vi "Butterfly_PullUp Capacitance AWG.vi"(0 "Semiconductor Module Context":T2, 2 "script name":string, 3 "C_TH_Delta":dbl=0.03 format="%#_13g", 4 "VNAs Measurement Parameters":T1, 5 "error in (no error)":errorcluster, 9 "Start_v":dbl=10.0 format="%#_13g", 11 "Stop_v":dbl=41.0 format="%#_13g") -> (14 "Semiconductor Module Context Out":T2, 19 "error out":errorcluster)   [LabVIEW 2013]
uses:
  <vilib>/NI_TestStand_SemiconductorModule/NI_TestStand_Semiconductor_Module.lvlibp/PinMap/General/SemiconductorModuleContext.ctl
  VNA/VNAs Measurement Parameters.ctl
  <instrlib>/niDCPower/nidcpower.llb/niDCPower Wait For Event - Event.ctl
  <instrlib>/niHSDIO/niHSDIO.llb/niHSDIO_ctl Trigger Script - trigID Values (Ring).ctl
  <vilib>/NI_TestStand_SemiconductorModule/NI_TestStand_Semiconductor_Module.lvlibp/PinMap/General/Publish/PublishDataDouble2D.vi
  <vilib>/NI_TestStand_SemiconductorModule/NI_TestStand_Semiconductor_Module.lvlibp
  VNA/Pin Map API/VNA Custom Instrument.lvlib
panel:
  out "Site":i32
  out "RL Step":i32
  out "PI Step":i32
  out "C_TH_PU":dbl format="%#_3g"
  out "C_Free":dbl[](array[numeric]) format="%#_3g"
  out "max index":i32
  out "BF C PI":dbl format="%#_3g"
  out "C_VPI":dbl
  out "BF C RL":dbl format="%#_3g"
  out "C_VRL":dbl
  out "appended array":dbl[][](array[numeric]) format="%#_3g"
  out "S3 steps":dbl[](array[numeric]) format="%#_3g"
  out "S2 steps":dbl[](array[numeric]) format="%#_3g"
  out "S1 steps":dbl[](array[numeric]) format="%#_3g"
  out "S0 steps":dbl[](array[numeric]) format="%#_3g"
  out "BF values":dbl[](array[numeric])
  out "VRLs":dbl[](array[numeric])
  out "VPIs":dbl[](array[numeric])
  out "Multisite Cap Data":dbl[][][](array[numeric])
  out "BF Names":string[](array[string])
  out "BFSamples":i32
  in  "Step_v":dbl=1.0
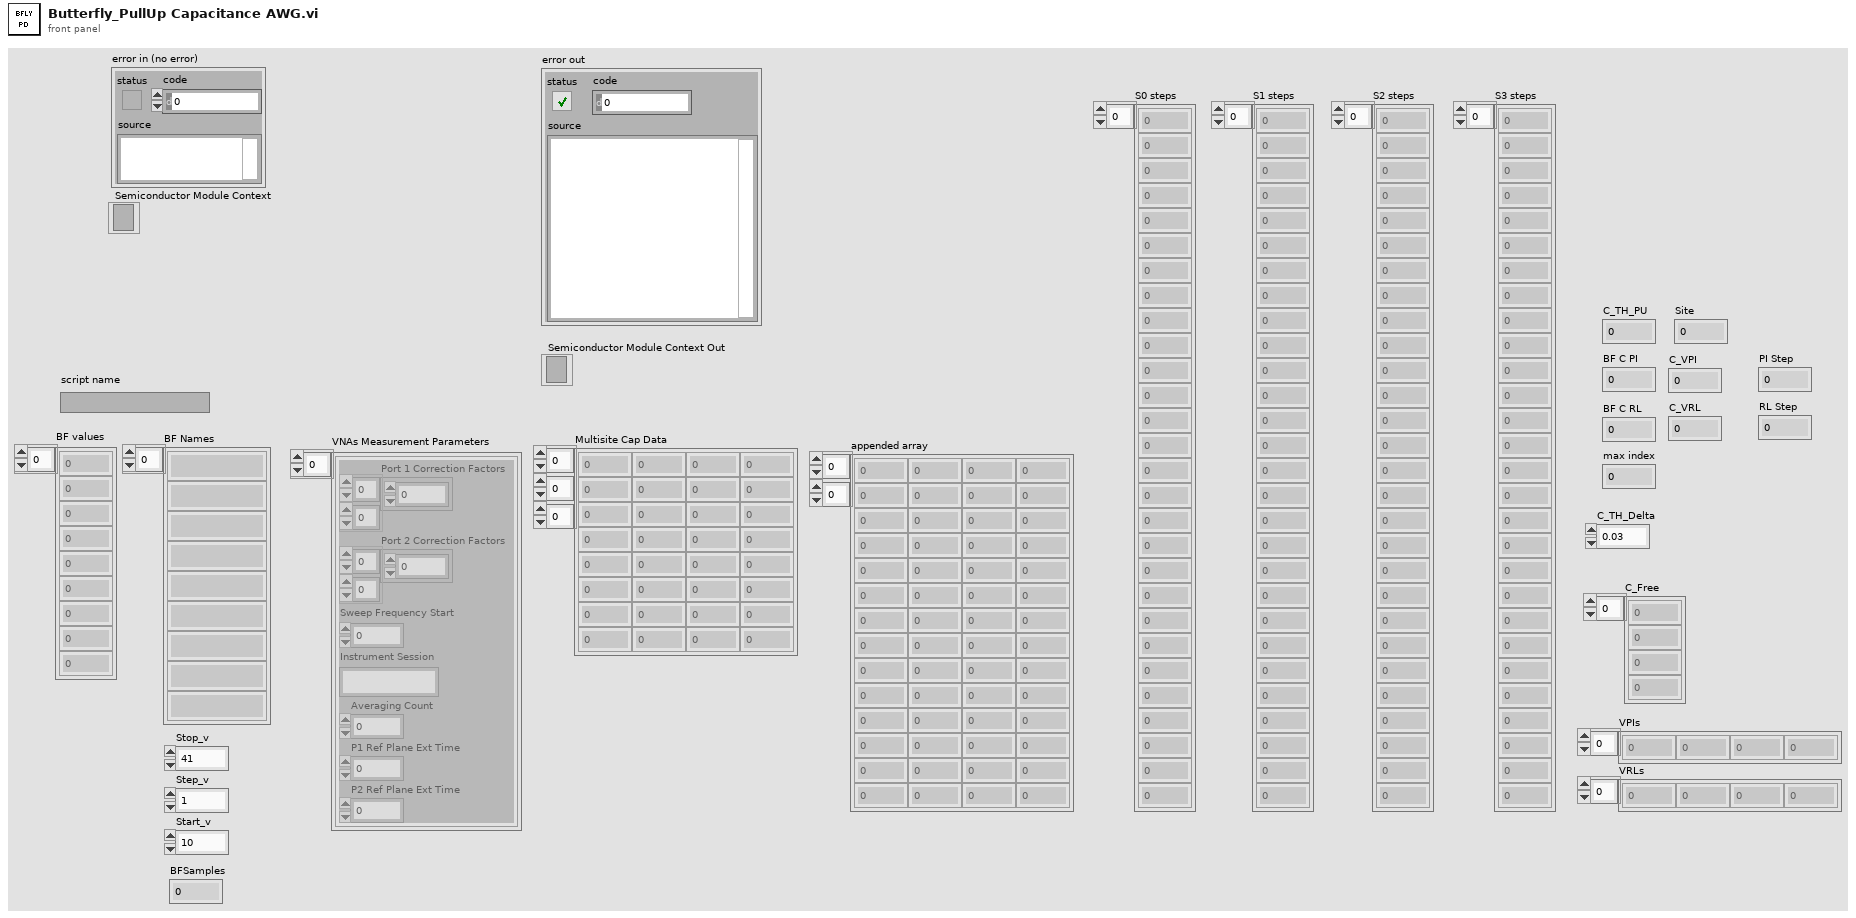
[diagram p1: front panel]
types:
  T1 = typedef "VNAs Measurement Parameters.ctl" = cluster{"Port 1 Correction Factors":cdb[][], "Port 2 Correction Factors":cdb[][], "Sweep Frequency Start":dbl, "Instrument Session":string, "Averaging Count":i32, "P1 Ref Plane Ext Time":dbl, "P2 Ref Plane Ext Time":dbl}[]
  T2 = typedef "NI_TestStand_Semiconductor_Module.lvlibp/SemiconductorModuleContext.ctl" = refnum<k7>
  T3 = typedef "niHSDIO_ctl Trigger Script - trigID Values (Ring).ctl" = string
  T4 = typedef "niDCPower Wait For Event - Event.ctl" = i32
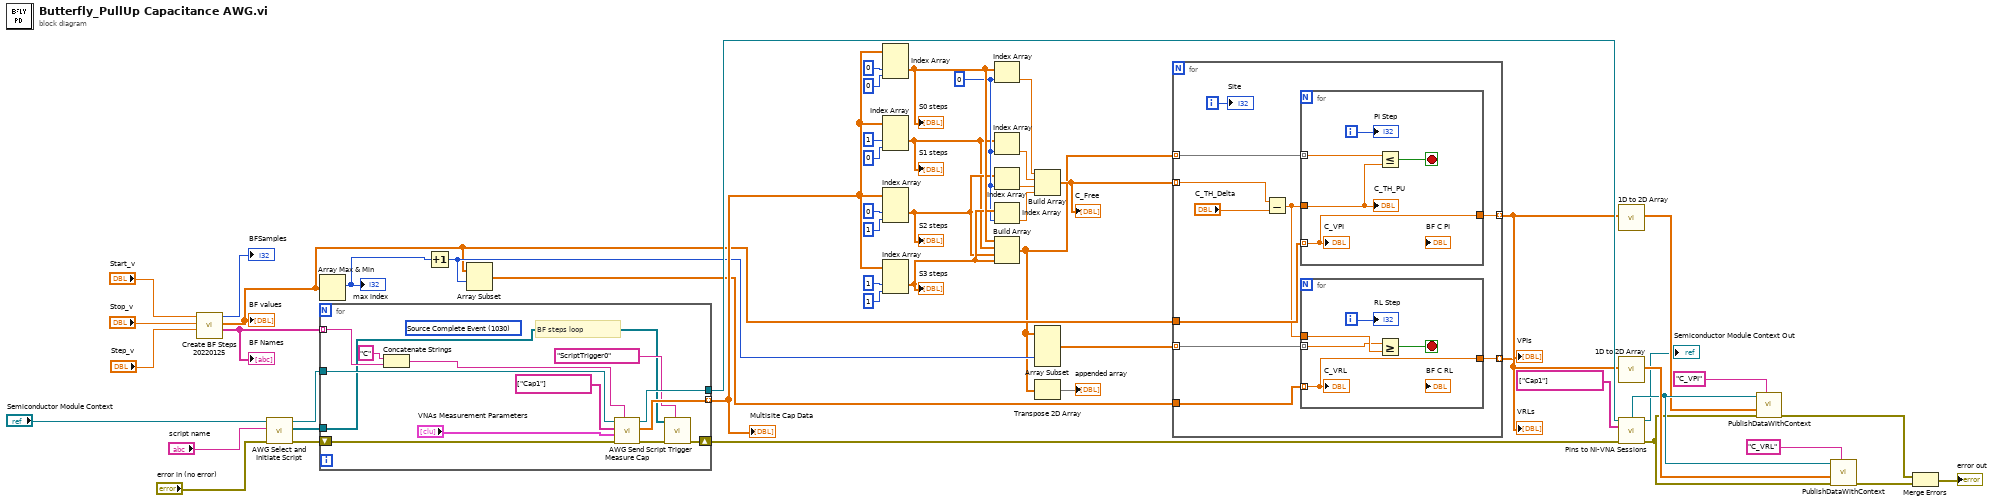
[diagram p0: block diagram]
diagram:
  w16 = 0 ("index")
  n1 = call "Create BF Steps 20220125.vi"("Step_v"="Step_v", "Stop_v"="Stop_v", "Start_v"="Start_v") -> ("BF Names"=w47:string[], "BF values"=w23:dbl[], "BFSamples"=→"BFSamples":i32)  [unwired: 6 in]
  "BF Names" <- w47
  "BF values" <- w23
  n2 = call "AWG Select and Initiate Script.vi"("error in (no error)"="error in (no error)", "script name"="script name", "Semiconductor Module Context"="Semiconductor Module Context") -> ("error out"=w2:errorcluster, "Sessions Out"=w6:refnum<k15>[], "Semiconductor Module Context Out"=w1:T2)  [unwired: 6 in]
  n3 = Array Max & Min(array=w23) -> (max index (indices)=w25:i32)  [unwired: 3 out]
  "max index" <- w25
  n4 = for {
    shift-right: [w55] -> w45
    shift-left: w2 -> [w57]
    tunnel: w1 -> [w62]
    tunnel: [w61] -> w52
    tunnel: [w60] -> w46 mode=indexing
    tunnel: w47 -> [w64] mode=indexing
    tunnel: w6 -> [w53]
    (unwired) T4 1030 items=["Source Complete Event"=1030, "Measure Complete Event"=1031, "Sequence Iteration Complete Event"=1032, "Sequence Engine Done Event"=1033, "Pulse Complete Event"=1051, "Ready For Pulse Trigger Event"=1052] ("event")
    # "BF steps loop"
    n5 = Concatenate Strings("C" ("string"), w64) -> (w63:string)
    n6 = call "Measure Cap.vi"("Measurement Id"=w63, "error in (no error)"=w57, "VNAs Measurement Parameters"="VNAs Measurement Parameters", "Pins"=string[] ["Cap1"] ("Capacitance Pins"), "Semiconductor Module Context"=w62) -> ("error out"=w56:errorcluster, "Multisite Cap Data"=w60:dbl[][], "Semiconductor Module Context Out"=w61:T2)  [unwired: 4 in]
    n7 = call "AWG Send Script Trigger.vi"("trigger id (script trigger 0)"=T3 "ScriptTrigger0", "error in (no error)"=w56, "AWG Sessions In"=w53) -> ("error out"=w55:errorcluster)  [unwired: 7 in, 1 out]
  }
  "Multisite Cap Data" <- w46
  n8 = Increment(x=w25) -> (x+1=w24:i32)
  n9 = Array Subset(array=w23, index=w24) -> (w22:dbl[])  [unwired: 1 in]
  n10 = Index Array(array=w46, index (dim 1)=0 ("disabled index (row)"), index (dim 2)=0 ("disabled index (col)")) -> (element=w19:dbl[])  [unwired: 1 in]
  "S0 steps" <- w19
  n11 = Index Array(array=w46, index (dim 1)=1 ("index (row)"), index (dim 2)=0 ("index (col)")) -> (element=w10:dbl[])  [unwired: 1 in]
  "S1 steps" <- w10
  n12 = Index Array(array=w46, index (dim 1)=0 ("index (row)"), index (dim 2)=1 ("index (col)")) -> (element=w11:dbl[])  [unwired: 1 in]
  "S2 steps" <- w11
  n13 = Index Array(array=w46, index (dim 1)=1 ("index (row)"), index (dim 2)=1 ("index (col)")) -> (element=w17:dbl[])  [unwired: 1 in]
  "S3 steps" <- w17
  n14 = Index Array(array=w19, index=w16) -> (element=w18:dbl)
  n15 = Index Array(array=w10, index=w16) -> (element=w15:dbl)
  n16 = Index Array(array=w11, index=w16) -> (element=w13:dbl)
  n17 = Index Array(array=w17, index=w16) -> (element=w14:dbl)
  n18 = Build Array(w19, w10, w11, w17) -> (w9:dbl[][])
  n19 = Build Array(w18, w15, w13, w14) -> (w12:dbl[])
  "C_Free" <- w12
  n20 = Array Subset(array=w9, index (col)=w24) -> (w26:dbl[][])  [unwired: 3 in]
  n21 = Transpose 2D Array(2D array=w9) -> (transposed array=→"appended array":dbl[][])
  n22 = for {
    tunnel: w23 -> [w75]
    tunnel: [w74] -> w21 mode=indexing
    tunnel: w22 -> [w73]
    tunnel: w26 -> [w72] mode=indexing
    tunnel: [w71] -> w20 mode=indexing
    tunnel: w12 -> [w68] mode=indexing
    tunnel: w9 -> [w69] mode=indexing
    i -> [w70]
    n23 = Subtract(x=w68, y="C_TH_Delta") -> (x-y=w66:dbl)
    n24 = for {
      tunnel: w75 -> [w84] mode=indexing
      tunnel: [w84] -> w74
      tunnel: w66 -> [w83]
      tunnel: w69 -> [w81] mode=indexing
      i -> [w82]
      stop <- w85 stop-if-true
      n25 = Less Or Equal?(x=w81, y=w83) -> (x <= y?=w85:bool)
      "C_VPI" <- w84
      "C_TH_PU" <- w83
      "PI Step" <- w82
    }
    n26 = for {
      tunnel: w73 -> [w79] mode=indexing
      tunnel: w72 -> [w76] mode=indexing
      tunnel: [w79] -> w71
      tunnel: w66 -> [w78]
      i -> [w77]
      stop <- w80 stop-if-true
      n27 = Greater Or Equal?(x=w76, y=w78) -> (x >= y?=w80:bool)
      "C_VRL" <- w79
      "RL Step" <- w77
    }
    "Site" <- w70
  }
  "VPIs" <- w21
  "VRLs" <- w20
  n28 = call "1D to 2D Array.vi"("1D Array"=w21) -> ("2D Array"=w30:dbl[][])  [unwired: 10 in]
  n29 = call "1D to 2D Array.vi"("1D Array"=w20) -> ("2D Array"=w43:dbl[][])  [unwired: 10 in]
  n30 = call "Pins to NI-VNA Sessions.vi"("Semiconductor Module Context"=w52, "Pins"=string[] ["Cap1"] ("Capacitance Pins"), "error in (no error)"=w45) -> ("Pin Query Context"=w31:refnum<class "MultiplePinMultipleSessionQueryContext.lvclass">, "Semiconductor Module Context Out"=→"Semiconductor Module Context Out":T2, "error out"=w27:errorcluster)  [unwired: 8 in, 2 out]
  n31 = call-poly <vilib>:"PublishDataWithContext.vi"("Published Data Id"="C_VPI", "error in (no error)"=w27, "Data In"=w30, "Pin Query Context"=w31) -> ("error out"=w28:errorcluster)  [unwired: 6 in, 1 out]
  n32 = call-poly <vilib>:"PublishDataWithContext.vi"("Published Data Id"="C_VRL", "error in (no error)"=w27, "Data In"=w43, "Pin Query Context"=w31) -> ("error out"=w44:errorcluster)  [unwired: 6 in, 1 out]
  n33 = Merge Errors(w28, w44) -> (→"error out":errorcluster)
